vi "readLine.vi"() -> ()   [LabVIEW 2010]
uses:
  <vilib>/rvi/interface/nirviMethod/nirviMethod.xnode
  <vilib>/rvi/interface/common/niFpgaNodeNameForErrorReporting.ctl
  <vilib>/rvi/errors/niLvFpgaWhatHappensToTopLevelVI.ctl
  <vilib>/Utility/error.llb/Error Cluster From Error Code.vi
  <vilib>/rvi/errors/niLvFpgaAdjustHostInterfaceError.vi
  NiFpgaLv.dll
panel:
  out "reader status out":T1
  out "error out":errorcluster
  in  "reader status":T1
  in  "error in":errorcluster
  in  "FPGA VI Reference In":refnum<k20>
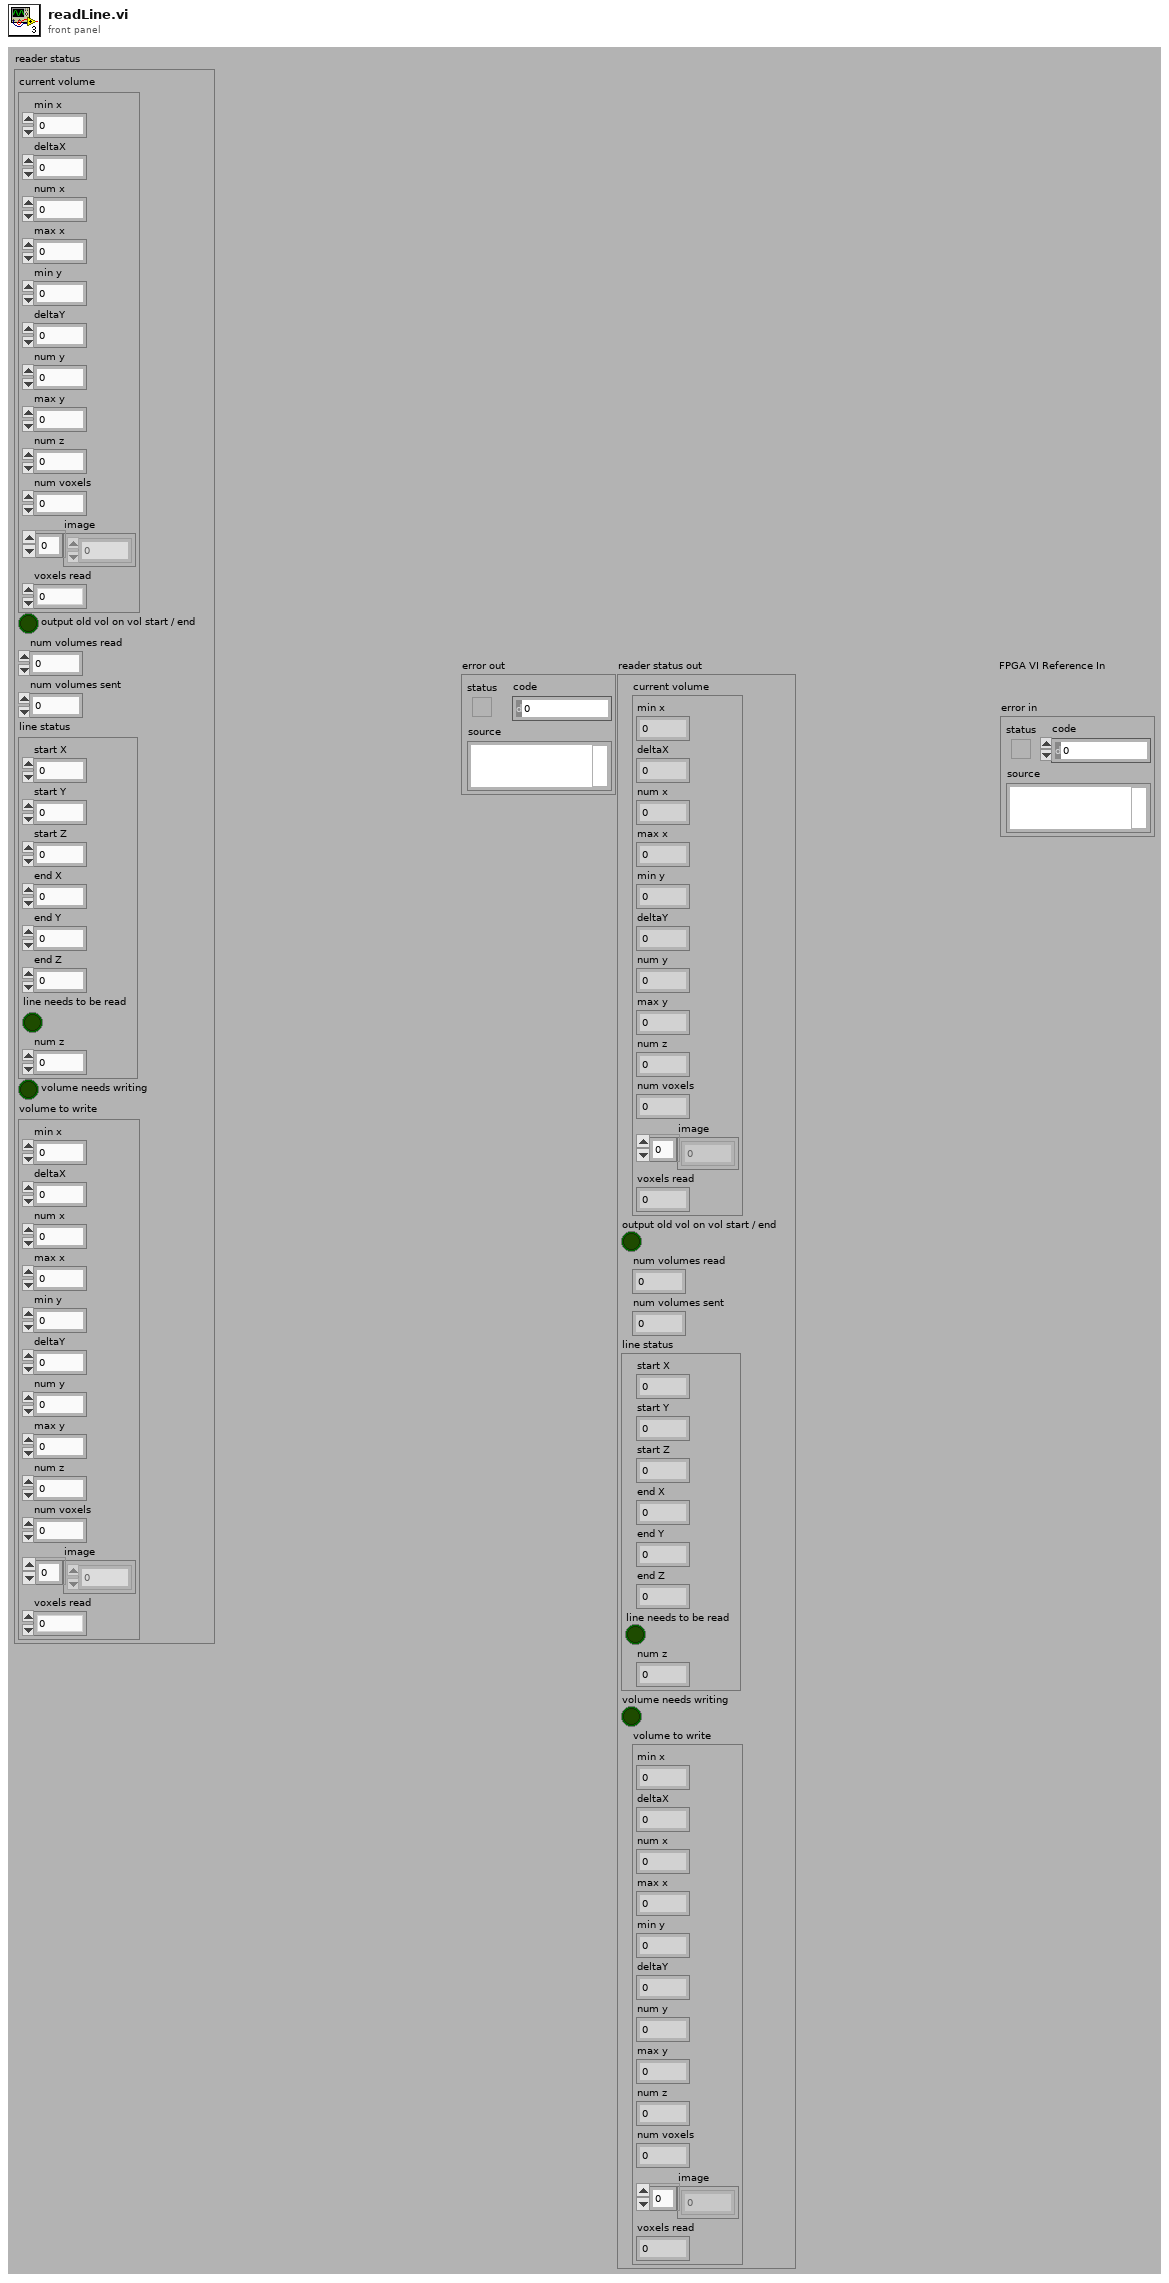
[diagram p1: front panel]
types:
  T1 = cluster{"current volume":cluster{"min x":i16, "deltaX":dbl, "num x":u32, "max x":i16, "min y":i16, "deltaY":dbl, "num y":u32, "max y":i16, "num z":u32, "num voxels":u32, "image":u32[], "voxels read":u32}, "output old vol on vol start / end":bool, "num volumes read":u32, "num volumes sent":u32, "line status":cluster{"start X":i16, "start Y":i16, "start Z":i16, "end X":i16, "end Y":i16, "end Z":i16, "line needs to be read":bool, "num z":u8}, "volume needs writing":bool, "volume to write":cluster{"min x":i16, "deltaX":dbl, "num x":u32, "max x":i16, "min y":i16, "deltaY":dbl, "num y":u32, "max y":i16, "num z":u32, "num voxels":u32, "image":u32[], "voxels read":u32}}
  T2 = typedef "niFpgaNodeNameForErrorReporting.ctl" = enum16{"Open FPGA VI Reference", "Read/Write Control", "Invoke Method: Abort", "Invoke Method: Acknowledge IRQ", "Invoke Method: Download", "Invoke Method: FIFO.Configure", "Invoke Method: FIFO.Read", "Invoke Method: FIFO.Start", "Invoke Method: FIFO.Stop", "Invoke Method: FIFO.Write", "Invoke Method: Reset", "Invoke Method: Run", "Invoke Method: Wait on IRQ", "Close FPGA VI Reference"}
  T3 = typedef "niLvFpgaWhatHappensToTopLevelVI.ctl" = enum16{"top level VI scripted behind XNode", "top level VI inlined behind XNode"}
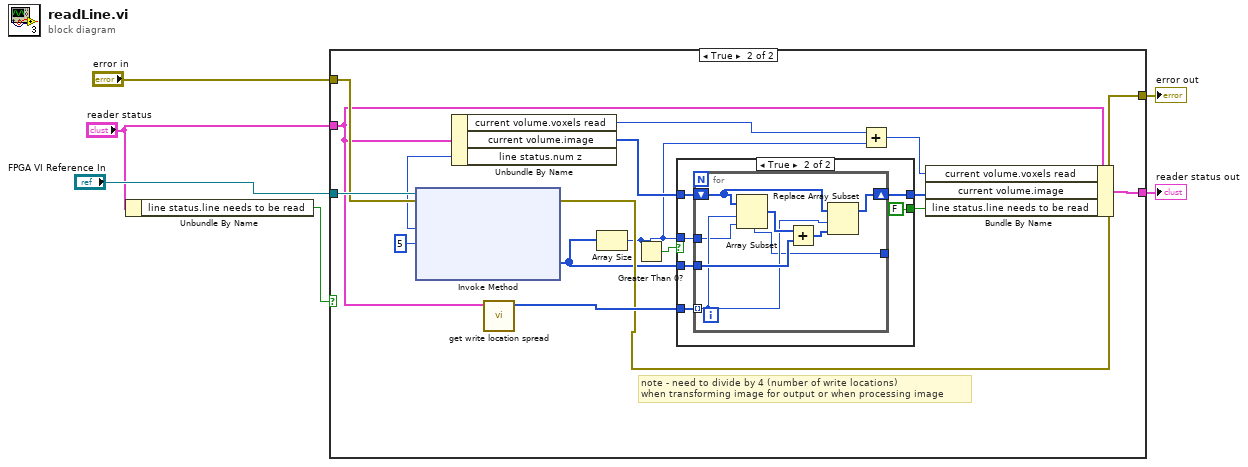
[diagram p0: block diagram]
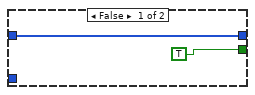
[diagram p3: hidden frame]
diagram:
  n1 = Unbundle By Name("reader status") -> ("line status.line needs to be read"=w4:bool)
  n2 = case shown="True" w4 {
    tunnel: "FPGA VI Reference In" -> [_ w24]
    tunnel: "error in" -> [w7 w23]
    tunnel: "reader status" -> [w8 w15]
    tunnel: [w8 w14] -> w1
    tunnel: [w7 w13] -> w2
    frame False {
    }
    frame True {
      # "note - need to divide by 4 (number of write locations)\nwhen transforming image for output or when processing image"
      n3 = Unbundle By Name(w15) -> ("current volume.voxels read"=w18:u32, "current volume.image"=w19:u32[], "line status.num z"=w22:u8)
      n4 = xnode "Invoke Method"("FPGA VI Reference In"=w24, "error in"=w23, "Number of Elements"=w22, "Timeout (ms)"=5) -> ("error out"=w13:errorcluster, "Data"=w12:u32[])  [unwired: 2 out]
      n5 = call "get write location spread.vi"("reader status"=w15) -> ("3D write locations"=w20:u32[])  [unwired: 9 in, 1 out]
      n6 = Array Size(array=w12) -> (size(s)=w10:i32)
      n7 = Greater Than 0?(x=w10) -> (x > 0?=w11:bool)
      n8 = case shown="True" w11 {
        tunnel: w20 -> [_ w32]
        tunnel: w19 -> [w26 w31]
        tunnel: [w26 w30] -> w17
        tunnel: w12 -> [_ w29]
        tunnel: w10 -> [_ w28]
        tunnel: [TRUE FALSE] -> w9
        frame False {
        }
        frame True {
          n9 = for {
            tunnel: w32 -> [w37] mode=indexing
            shift-right: [w34] -> w30
            shift-left: w31 -> [w36]
            tunnel: w29 -> [w38]
            tunnel: [w33] -> _
            tunnel: w28 -> [w33]
            n10 = Array Subset(array=w36, index=w37, length=w33) -> (w39:u32[])
            n11 = Add(x=w39, y=w38) -> (x+y=w35:u32[])
            n12 = Replace Array Subset(array=w36, new element=w35, index=w37) -> (w34:u32[])
          }
        }
      }
      n13 = Add(x=w18, y=w10) -> (x+y=w16:u32)
      n14 = Bundle By Name(cluster=w15, "current volume.voxels read"=w16, "current volume.image"=w17, "line status.line needs to be read"=w9) -> (w14:T1)
    }
  }
  "error out" <- w2
  "reader status out" <- w1
